vi "Record_Frame.vi"(8 "error in":errorcluster, 9 "Settings":T6={"Harware Configuration"={"Camera"="cam1", "Frames Per Second"=15, "Simulate Recording"=FALSE, "Simulated Recording Sample"=path "", "Timestamp Method"=enum."Camera Timestamp"}, "Base Recording Path"=path "", "Type Of Recording"="", "Recording Codec"="", "TrackingSettings"={"Max Radius"=0, "Threshold"=160.0, "ROI"={"Left"=0, "Top"=0, "Right"=0, "Bottom"=0, "Rotation"=0.0}}, "Calibration"={"Pixel Width (X)"=1.0, "Pixel Height (Y)"=1.0}, "Broadcast Length"=0} {"Broadcast Length" min=0; "TrackingSettings"."ROI"."Rotation" format="%.2f"; "TrackingSettings"."ROI"."Left" scale=0.0..1024.0; "TrackingSettings"."ROI"."Right" scale=0.0..1024.0; "TrackingSettings"."Threshold" scale=0.0..255.0}, 10 "Image Data":T1 {"Frame Data"."Image Type" items=["Grayscale (U8)", "Grayscale (I16)", "Grayscale (SGL)", "Complex (CSG)", "RGB (U32)", "HSL (U32)", "RGB (U64)", "Grayscale (U16)"]}, 11 "Recording Data In":T3) -> (0 "error out":errorcluster, 3 "Recording Data Out":T3)   [LabVIEW 2017, in "ImageAcquisitionLibrary.lvlib"]
uses:
  ImageAcquisitionLibrary.lvlib
  Settings/Settings.ctl
  <vilib>/userdefined/High Color/IMAQdx.ctl
  Tracking/TrackingSettings.ctl
  Settings/Calibration.ctl
  RecordingData.ctl
  <vilib>/vision/Image Controls.llb/IMAQ Image.ctl
  <vilib>/vision/Avi.llb/IMAQ AVI2 Refnum.ctl
  Acquisition/AcquireData.ctl
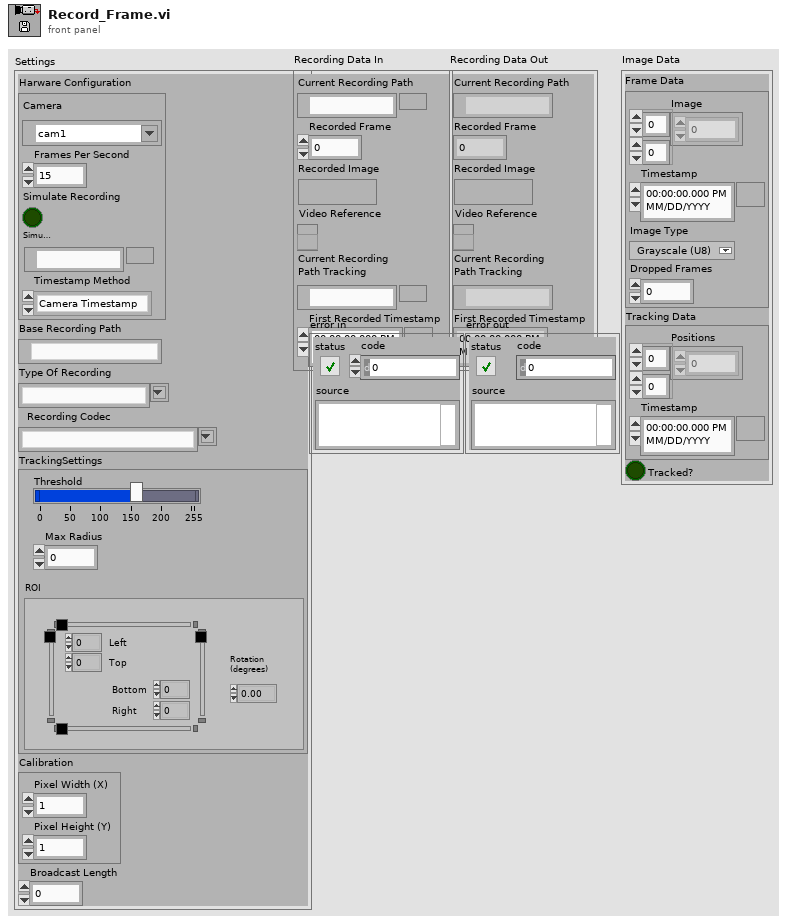
[diagram p1: front panel]
types:
  T1 = typedef "ImageAcquisitionLibrary.lvlib/AcquireData.ctl" = cluster{"Frame Data":cluster{"Image":u32[][], "Timestamp":timestamp, "Image Type":T2, "Dropped Frames":u32}, "Tracking Data":cluster{"Positions":dbl[][], "Timestamp":timestamp}, "Tracked?":bool}
  T2 = typedef "Image Type" = u32
  T3 = typedef "ImageAcquisitionLibrary.lvlib/RecordingData.ctl" = cluster{"Current Recording Path":path, "Recorded Frame":i32, "Recorded Image":T4, "Video Reference":T5, "Current Recording \nPath Tracking":path, "First Recorded Timestamp":timestamp}
  T4 = typedef "IMAQ Image.ctl" = refnum<image>
  T5 = typedef "IMAQ AVI2 Refnum.ctl" = refnum<k20>
  T6 = typedef "ImageAcquisitionLibrary.lvlib/Settings.ctl" = cluster{"Harware Configuration":cluster{"Camera":T7, "Frames Per Second":u32, "Simulate Recording":bool, "Simulated Recording Sample":path, "Timestamp Method":enum16{"System Timestamp", "Camera Timestamp", "IMAQdx Timestamp"}}, "Base Recording Path":path, "Type Of Recording":string, "Recording Codec":string, "TrackingSettings":T8, "Calibration":T10, "Broadcast Length":i32}
  T7 = typedef "IMAQdx.ctl" = refnum<k21>
  T8 = typedef "ImageAcquisitionLibrary.lvlib/TrackingSettings.ctl" = cluster{"Max Radius":i32, "Threshold":sgl, "ROI":T9}
  T9 = typedef "IMAQ Rectangle" = cluster{"Left":i32, "Top":i32, "Right":i32, "Bottom":i32, "Rotation":dbl}
  T10 = typedef "ImageAcquisitionLibrary.lvlib/Calibration.ctl" = cluster{"Pixel Width (X)":dbl, "Pixel Height (Y)":dbl}
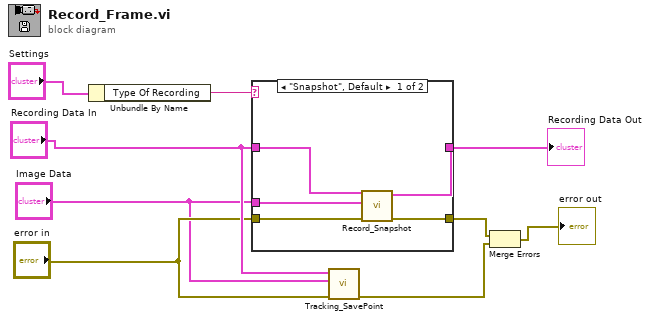
[diagram p0: block diagram]
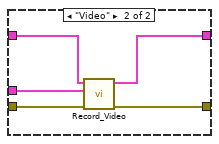
[diagram p2: hidden frame]
diagram:
  n1 = Unbundle By Name("Settings") -> ("Type Of Recording"=w9:string)
  n2 = case shown="\"Snapshot\", Default" w9 {
    tunnel: "Image Data" -> [w11 w17]
    tunnel: "Recording Data In" -> [w10 w16]
    tunnel: "error in" -> [w14 w19]
    tunnel: [w13 w18] -> w5
    tunnel: [w12 w15] -> w7
    frame "Snapshot", Default {
      n3 = call "Record_Snapshot.vi"("error in (no error)"=w14, "Data In"=w11, "Recording Data"=w10) -> ("error out"=w13:errorcluster, "Recording Data Out"=w12:T3)  [unwired: 7 in]
    }
    frame "Video" {
      n4 = call "Record_Video.vi"("error in (no error)"=w19, "Data In"=w17, "Recording Data In"=w16) -> ("error out"=w18:errorcluster, "Recording Data Out"=w15:T3)  [unwired: 7 in]
    }
  }
  "Recording Data Out" <- w7
  n5 = call "Tracking_SavePoint.vi"("error in"="error in", "Image Data"="Image Data", "Recording Data In"="Recording Data In") -> ("error out"=w4:errorcluster)  [unwired: 8 in]
  n6 = Merge Errors(w5, w4) -> (→"error out":errorcluster)
